vi "Arrange VIWin - Arrange FP.vi"(0 "VI in":refnum<vi>, 11 "error in":errorcluster) -> (15 "error out":errorcluster)   [LabVIEW 2020, in "Arrange VI Window.lvlib"]
uses:
  Arrange VI Window.lvlib
  Arrange VIWin - Window Type.ctl
  <vilib>/Utility/miscctls.llb/LVPointTypeDef.ctl
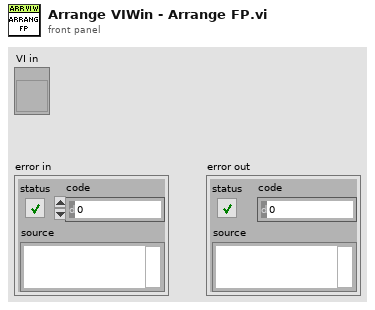
[diagram p1: front panel]
types:
  T1 = typedef "Arrange VI Window.lvlib/Arrange VIWin - Window Type.ctl" = enum16{"FP", "BD"}
  T2 = typedef "LVPointTypeDef.ctl" = cluster{"Horizontal":i16, "Vertical":i16}
  T3 = typedef "LVRectTypeDef.ctl" = cluster{"Left":i16, "Top":i16, "Right":i16, "Bottom":i16}
  T4 = typedef "Arrange VI Window.lvlib/Arrange VIWin - Min Window Dimensions.ctl" = cluster{"min window width":i16, "min window height":i16}
  T5 = typedef "Arrange VI Window.lvlib/Arrange VIWin - Window Gaps.ctl" = cluster{"left gap":i16, "top gap":i16, "min right gap":i16, "min bottom gap":i16}
  T6 = cluster{"display workspace bounds":T3, "min window dimensions":T4, "window gaps":T5}
  T7 = typedef "Arrange VI Window.lvlib/Arrange VIWin - FP Objects Arrangement Info.ctl" = cluster{"grid size":i32, "horizontal margin factor":i32, "horizontal spacing factor":i32, "vertical margin factor":i32, "vertical spacing factor":i32}
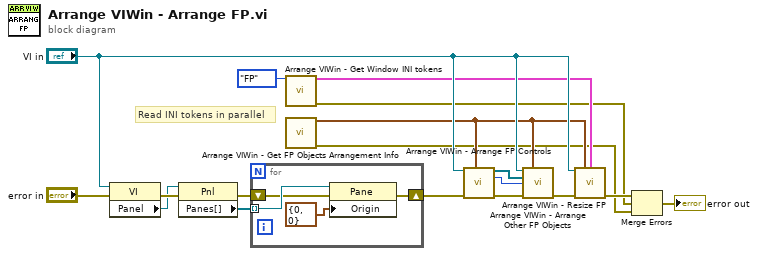
[diagram p0: block diagram]
diagram:
  # "Read INI tokens in parallel"
  n1 = property class="VI"(reference="VI in", error in="error in") -> (error out=w15:errorcluster, "Panel"=w14:refnum<vi>)  [unwired: 1 out]
  n2 = property class="Pnl"(reference=w14, error in=w15) -> (error out=w16:errorcluster, "Panes[]"=w17:refnum<vi>[])  [unwired: 1 out]
  n3 = for {
    tunnel: w17 -> [w22] mode=indexing
    shift-right: [w20] -> w6
    shift-left: w16 -> [w21]
    n4 = property class="Pane"(reference=w22, error in=w21, "Origin"=T2 {"Horizontal"=0, "Vertical"=0}) -> (error out=w20:errorcluster)  [unwired: 1 out]
  }
  n5 = call "Arrange VIWin - Get Window INI tokens.vi"("window type"=Arrange_VIWin_-_Window_Type."FP") -> ("Window INI tokens"=w5:T6, "error out"=w2:errorcluster)  [unwired: 13 in]
  n6 = call "Arrange VIWin - Get FP Objects Arrangement Info.vi"() -> ("FP objects arrangement info"=w9:T7, "error out"=w1:errorcluster)  [unwired: 14 in]
  n7 = call "Arrange VIWin - Arrange FP Controls.vi"("VI in"="VI in", "FP objects arrangement info"=w9, "error in"=w6) -> ("controls from conn pane"=w11:refnum<vi>[], "max bottom"=w10:i16, "error out"=w18:errorcluster)  [unwired: 10 in]
  n8 = call "Arrange VIWin - Arrange Other FP Objects.vi"("VI in"="VI in", "FP objects arrangement info"=w9, "controls from conn pane"=w11, "max bottom of arranged controls"=w10, "error in"=w18) -> ("error out"=w13:errorcluster)  [unwired: 10 in]
  n9 = call "Arrange VIWin - Resize FP.vi"("VI in"="VI in", "FP objects arrangement info"=w9, "Window INI tokens"=w5, "error in"=w13) -> ("error out"=w7:errorcluster)  [unwired: 11 in]
  n10 = Merge Errors(w7, w2, w1) -> (→"error out":errorcluster)
